vi "Polynomkoeffizienten.vi"() -> ()   [LabVIEW 2015, in "Linearisierung V2.lvlib"]
uses:
  Linearisierung V2.lvlib
  Visualisierungs Elemente/Button.ctl
  Visualisierungs Elemente/String - Ausgabefeld.ctl
  Aktionen Polynom Daten speichern.ctl
  Seiten/FT-IR/FGV FT-IR Gasliste Aktionen.ctl
  Passwortverwaltung/FGV Passwort Aktion.ctl
  Seiten/FT-IR/FT-IR.lvlib
  Passwortverwaltung/Passwort.lvlib
  Allgemein/allgemeine Sub-VIs.lvlib
  Sprachverwaltung/Sprachverwaltung.lvlib
panel:
  in  "Auf":T1
  in  "Ab":T1
  out "Namen":string[](array[string])
  out "Aktuelle Gasliste":T2[](array[typedef])
  in  "Aktiv":bool[](array[boolean])
  in  "Speichern":T1
  in  "ABBRECHEN":T1
  in  "Polynome":sgl[][](array[numeric])
  # "Polynomkoeffizienten"
  # "Gasliste"
  # "Namen"
  # "Polynomkoeffizienten"
  # "AKTIV"
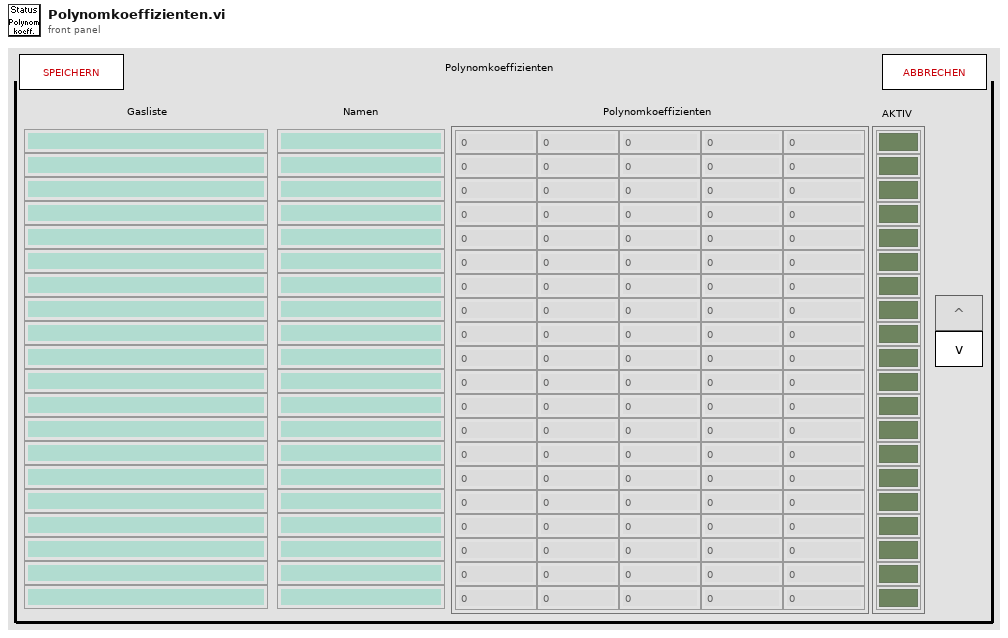
[diagram p1: front panel]
types:
  T1 = typedef "Button.ctl" = bool
  T2 = typedef "String - Ausgabefeld.ctl" = string
  T3 = enum8{"Enabled", "Disabled", "Disabled and Grayed Out"}
  T4 = typedef "FT-IR.lvlib/FGV FT-IR Gasliste Aktionen.ctl" = enum16{"lesen", "Gasliste FT-IR", "Gasliste ausgelesen", "laden", "speichern", "löschen"}
  T5 = typedef "Linearisierung V2.lvlib/Aktionen Polynom Daten speichern.ctl" = enum16{"lesen", "laden", "speichern", "schreiben1", "schreiben alle", "Liste erstellen"}
  T6 = typedef "Passwort.lvlib/FGV Passwort Aktion.ctl" = enum16{"prüfen", "setzen", "Initialisieren", "PW speichern", "lesen", "PW Änderung"}
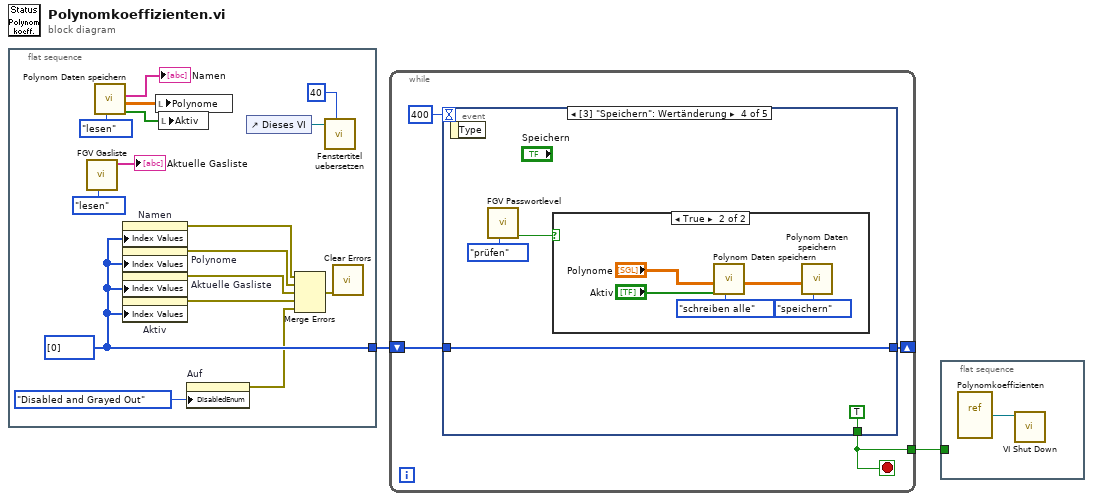
[diagram p0: block diagram]
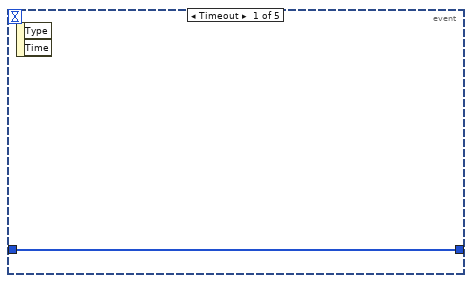
[diagram p2: hidden frame]
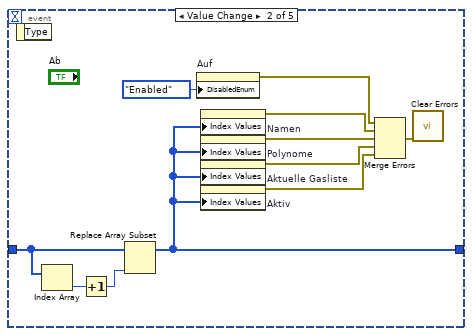
[diagram p3: hidden frame]
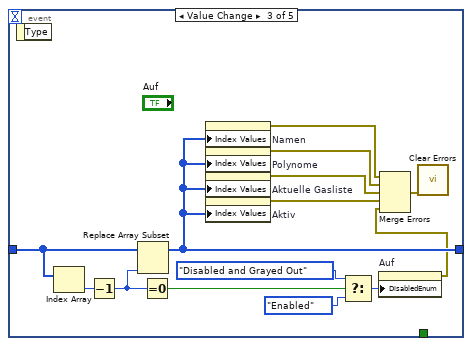
[diagram p4: hidden frame]
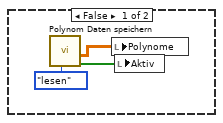
[diagram p5: hidden frame]
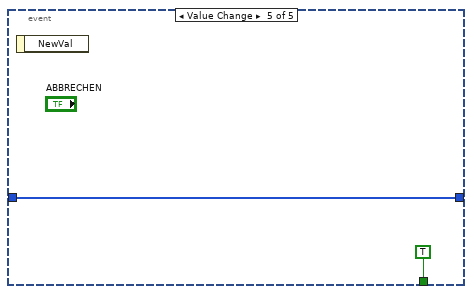
[diagram p6: hidden frame]
diagram:
  n1 = flat-sequence {
    tunnel: [w11] -> w1
    frame #0 {
      w11 = u32[] [0] ("Indexwerte")
      n2 = call "FGV Gasliste.vi"("Aktionen"=FGV_FT-IR_Gasliste_Aktionen."lesen") -> ("Aktuelle Gasliste FT-IR"=→"Aktuelle Gasliste":T2[])  [unwired: 8 in, 2 out]
      n3 = call "Polynom Daten speichern.vi"("Aktionen"=Aktionen_Polynom_Daten_speichern."lesen") -> ("Aktiv"=w15:bool[], "Polynome"=w13:sgl[][], "Namen"=→"Namen":string[])  [unwired: 7 in, 1 out]
      n4 = property on="Namen" class="Arr (strikt)"("Index Values"=w11) -> (error out=w10:errorcluster)  [unwired: 2 in, 1 out]
      n5 = property on="Polynome" class="Arr (strikt)"("Index Values"=w11) -> (error out=w9:errorcluster)  [unwired: 2 in, 1 out]
      n6 = property on="Aktuelle Gasliste" class="Arr (strikt)"("Index Values"=w11) -> (error out=w8:errorcluster)  [unwired: 2 in, 1 out]
      n7 = property on="Aktiv" class="Arr (strikt)"("Index Values"=w11) -> (error out=w7:errorcluster)  [unwired: 2 in, 1 out]
      n8 = local write "Polynome"(w13) -> ()
      n9 = local write "Aktiv"(w15) -> ()
      n10 = property on="Auf" class="Bool."("DisabledEnum"=T3."Disabled and Grayed Out" ("t")) -> (error out=w6:errorcluster)  [unwired: 2 in, 1 out]
      n11 = control-ref of="Dieses VI"() -> (w4:refnum<vi>)
      n12 = Merge Errors(w10, w9, w8, w7, w6) -> (w5:errorcluster)
      n13 = call "Fenstertitel uebersetzen.vi"("Index (Seite)"=40, "Dieses VI"=w4) -> ()  [unwired: 8 in, 2 out]
      n14 = call <vilib>:"Clear Errors.vi"("error in (no error)"=w5) -> ()  [unwired: 5 in, 2 out]
    }
  }
  n15 = while {
    tunnel: [w21] -> w2
    shift-right: [w19] -> _
    shift-left: w1 -> [w20]
    stop <- w21 stop-if-true
    n16 = event shown="[3] \"Speichern\": Wertänderung" {
      selector: _ -> [_ _ _ _ _]
      dyn-events: _ -> [_ _ _ _ _]
      timeout: 400 -> [_ _ _ _ _]
      tunnel: [_ _ _ TRUE ("ABBRECHEN") TRUE ("ABBRECHEN")] -> w21
      tunnel: w20 -> [w23 w33 w47 w51 w61]
      tunnel: [w23 w30 w41 w51 w61] -> w19
      event Timeout {
        n17 = event-data() -> ()  [unwired: 1 in, 2 out]
      }
      event Value Change {
        n18 = event-data() -> ()  [unwired: 1 in, 1 out]
        n19 = Index Array(array=w33) -> (element=w34:u32)  [unwired: 1 in]
        n20 = Increment(x=w34) -> (x+1=w32:u32)
        n21 = Replace Array Subset(array=w33, new element=w32) -> (w30:u32[])  [unwired: 1 in]
        n22 = property on="Auf" class="Bool."("DisabledEnum"=T3."Enabled" ("t")) -> (error out=w28:errorcluster)  [unwired: 2 in, 1 out]
        n23 = property on="Namen" class="Arr (strikt)"("Index Values"=w30) -> (error out=w27:errorcluster)  [unwired: 2 in, 1 out]
        n24 = property on="Polynome" class="Arr (strikt)"("Index Values"=w30) -> (error out=w26:errorcluster)  [unwired: 2 in, 1 out]
        n25 = property on="Aktuelle Gasliste" class="Arr (strikt)"("Index Values"=w30) -> (error out=w25:errorcluster)  [unwired: 2 in, 1 out]
        n26 = property on="Aktiv" class="Arr (strikt)"("Index Values"=w30) -> (error out=w24:errorcluster)  [unwired: 2 in, 1 out]
        n27 = Merge Errors(w28, w27, w26, w25, w24) -> (w29:errorcluster)
        n28 = call <vilib>:"Clear Errors.vi"("error in (no error)"=w29) -> ()  [unwired: 5 in, 2 out]
      }
      event Value Change {
        n29 = event-data() -> ()  [unwired: 1 in, 1 out]
        n30 = Index Array(array=w47) -> (element=w48:u32)  [unwired: 1 in]
        n31 = Decrement(x=w48) -> (x-1=w46:u32)
        n32 = Replace Array Subset(array=w47, new element=w46) -> (w41:u32[])  [unwired: 1 in]
        n33 = Equal To 0?(x=w46) -> (x = 0?=w42:bool)
        n34 = property on="Namen" class="Arr (strikt)"("Index Values"=w41) -> (error out=w39:errorcluster)  [unwired: 2 in, 1 out]
        n35 = property on="Polynome" class="Arr (strikt)"("Index Values"=w41) -> (error out=w38:errorcluster)  [unwired: 2 in, 1 out]
        n36 = property on="Aktuelle Gasliste" class="Arr (strikt)"("Index Values"=w41) -> (error out=w37:errorcluster)  [unwired: 2 in, 1 out]
        n37 = property on="Aktiv" class="Arr (strikt)"("Index Values"=w41) -> (error out=w36:errorcluster)  [unwired: 2 in, 1 out]
        n38 = Select(t=T3."Disabled and Grayed Out", s=w42, f=T3."Enabled" ("Deaktiviert")) -> (s? t:f=w44:T3)
        n39 = property on="Auf" class="Bool."("DisabledEnum"=w44) -> (error out=w35:errorcluster)  [unwired: 2 in, 1 out]
        n40 = Merge Errors(w39, w38, w37, w36, w35) -> (w40:errorcluster)
        n41 = call <vilib>:"Clear Errors.vi"("error in (no error)"=w40) -> ()  [unwired: 5 in, 2 out]
      }
      event Value Change {
        n42 = event-data() -> ()  [unwired: 1 in, 1 out]
        n43 = call "FGV Passwortlevel.vi"("FGV Passwort Aktion"=FGV_Passwort_Aktion."prüfen") -> ("Freigabe"=w49:bool)  [unwired: 8 in, 2 out]
        n44 = case shown="True" w49 {
          frame False {
            n45 = call "Polynom Daten speichern.vi"("Aktionen"=Aktionen_Polynom_Daten_speichern."lesen") -> ("Aktiv"=w53:bool[], "Polynome"=w54:sgl[][])  [unwired: 7 in, 2 out]
            n46 = local write "Polynome"(w54) -> ()
            n47 = local write "Aktiv"(w53) -> ()
          }
          frame True {
            n48 = call "Polynom Daten speichern.vi"("Aktionen"=Aktionen_Polynom_Daten_speichern."schreiben alle", "Aktiv"="Aktiv", "Polynome"="Polynome") -> ("Polynome"=w56:sgl[][])  [unwired: 5 in, 3 out]
            n49 = call "Polynom Daten speichern.vi"("Aktionen"=Aktionen_Polynom_Daten_speichern."speichern", "Polynome"=w56) -> ()  [unwired: 6 in, 4 out]
          }
        }
      }
      event Value Change {
        n50 = event-data() -> ()  [unwired: 1 in, 1 out]
      }
    }
  }
  n51 = flat-sequence {
    tunnel: w2 -> [_]
    frame #0 {
      n52 = vi-ref "Polynomkoeffizienten.vi"() -> (w63:refnum<vi>)
      n53 = call "VI Shut Down.vi"("VI Referenz"=w63) -> ()  [unwired: 11 in]
    }
  }
